vi "Add.vi"(8 "error in (no error)":errorcluster, 9 "Value":variant, 10 "Key":variant, 11 "Store in":refnum<class "Store.lvclass">) -> (0 "error out":errorcluster, 1 "Success?":bool, 3 "Store out":refnum<class "Store.lvclass">)   [LabVIEW 2018, in "Application.lvlib" / "Store.lvclass"]
uses:
  Store.lvclass
  Store.lvclass/Store.ctl
  Dictionary Class/Dictionary.lvclass/Dictionary.ctl
  e194419b-6248-448c-bfd0-3bb9f5219d49.vi
  Dictionary Class/VIs/Get Data DVR.vi
  Variant to Packed String.vi
  Dictionary Class/Dictionary.lvclass
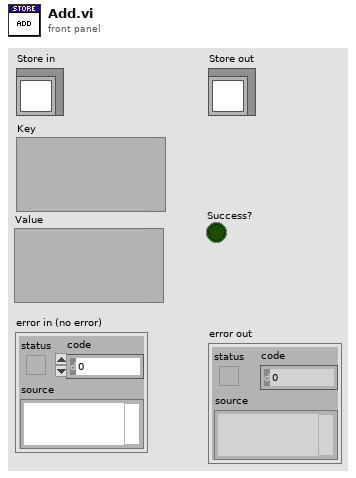
[diagram p1: front panel]
types:
  T1 = typedef "Application.lvlib/Store.lvclass/Packet.ctl" = cluster{"Type Descriptor":i16[], "Value":variant}
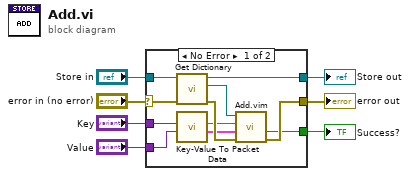
[diagram p0: block diagram]
diagram:
  n1 = case shown="No Error" "error in (no error)" {
    selector: "error in (no error)" -> [w13 w20]
    tunnel: [w9 w20] -> w6
    tunnel: [w14 w19] -> w4
    tunnel: "Store in" -> [w18 w19]
    tunnel: "Key" -> [w16 _]
    tunnel: "Value" -> [w15 _]
    tunnel: [w8 _] -> w1
    frame No Error {
      n2 = call "Get Dictionary.vi"("error in (no error)"=w13, "Store in"=w18) -> ("error out"=w12:errorcluster, "Dictionary.lvclass"=w17:refnum<class "Dictionary.lvclass">, "Store out"=w14:refnum<class "Store.lvclass">)  [unwired: 7 in]
      n3 = call "Key-Value To Packet Data.vi"("Value"=w15, "Key"=w16) -> ("Packet"=w10:T1, "Packed String"=w11:string)  [unwired: 8 in]
      n4 = call "Add.vim"("error in (no error)"=w12, "Value"=w10, "Key"=w11, "Dictionary in"=w17) -> ("error out"=w9:errorcluster, "Success?"=w8:bool)  [unwired: 5 in, 1 out]
    }
    frame Error {
    }
  }
  "error out" <- w6
  "Store out" <- w4
  "Success?" <- w1
